vi "manifold config control duplicate check (sub-vi).vi"(10 "manifold config array":T1) -> (2 "manifold config error flag array":bool[][](array[boolean]))   [LabVIEW 2021]
uses:
  type-defs/manifold configuration cluster array (type def).ctl
  type-defs/manifold configuration cluster (type def).ctl
  type-defs/manifold selection.ctl
  type-defs/single port single odor cluster.ctl
  type-defs/port number (type def).ctl
  type-defs/odor selection (type def).ctl
  type-defs/odor color (type def).ctl
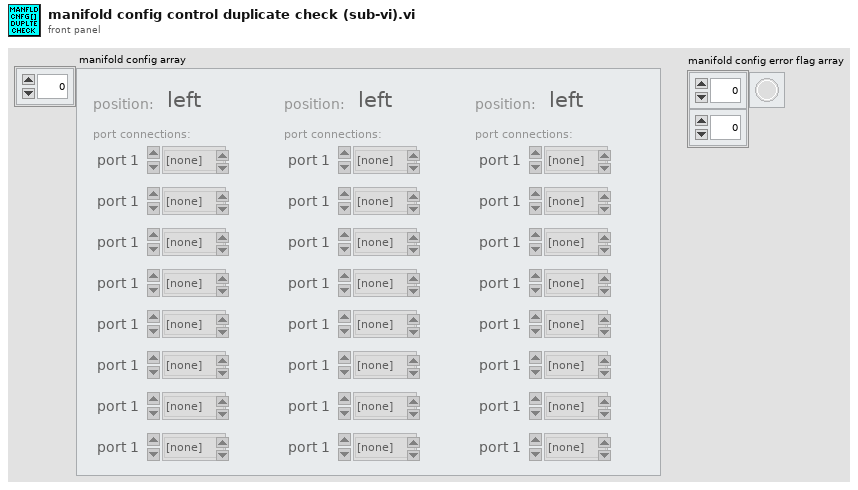
[diagram p1: front panel]
types:
  T1 = typedef "manifold configuration cluster array (type def).ctl" = T2[]
  T2 = typedef "manifold configuration cluster (type def).ctl" = cluster{"position:":T3, "port connections:":T4[]}
  T3 = typedef "manifold selection.ctl" = enum16{"left", "middle", "right"}
  T4 = typedef "single port single odor cluster.ctl" = cluster{"port number":T5, "connected odor":T6, "error":bool, "odor color":T7}
  T5 = typedef "port number (type def).ctl" = enum16{"port 1", "port 2", "port 3", "port 4", "port 5", "port 6", "port 7", "port 8"}
  T6 = typedef "odor selection (type def).ctl" = enum16{"[none]", "odor 1", "odor 2", "odor 3", "odor 4", "odor 5", "odor 6", "odor 7", "odor 8", "odor 9", "odor 10"}
  T7 = typedef "odor color (type def).ctl" = u16
  T8 = typedef "odor channel to odor count map (type def).ctl" = map{T6, u16}
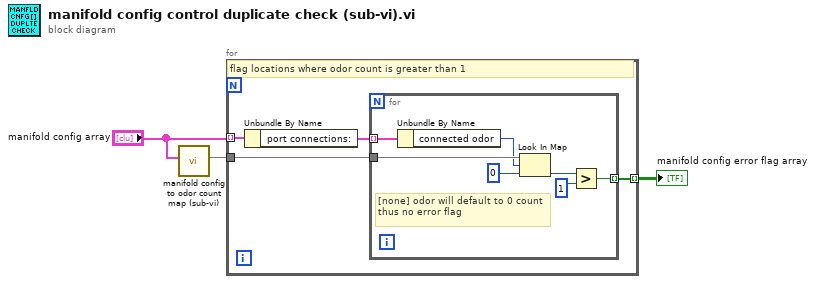
[diagram p0: block diagram]
diagram:
  n1 = call "manifold config to odor count map (sub-vi).vi"("manifold config array"="manifold config array") -> ("odor count map"=w2:T8)  [unwired: 10 in]
  n2 = for {
    tunnel: "manifold config array" -> [w7] mode=indexing
    tunnel: [w5] -> w1 mode=indexing
    tunnel: w2 -> [w4]
    # "flag locations where odor count is greater than 1"
    n3 = Unbundle By Name(w7) -> ("port connections:"=w6:T4[])
    n4 = for {
      tunnel: w6 -> [w14] mode=indexing
      tunnel: [w11] -> w5 mode=indexing
      tunnel: w4 -> [w9]
      # "[none] odor will default to 0 count\nthus no error flag"
      n5 = Unbundle By Name(w14) -> ("connected odor"=w8:T6)
      n6 = Look In Map(map=w9, key=w8, default value=u16 0) -> (value=w13:u16)  [unwired: 1 out]
      n7 = Greater?(x=w13, y=u16 1) -> (0:w11:bool)
    }
  }
  "manifold config error flag array" <- w1
